vi "Read Number of Crossover Points.vi"(8 "error in (no error)":errorcluster, 11 "N-Point Crossover in":refnum<class "N-Point Crossover.lvclass">) -> (0 "error out":errorcluster, 2 "X-Point":T1, 3 "N-Point Crossover out":refnum<class "N-Point Crossover.lvclass">)   [LabVIEW 2016, in "N-Point Crossover.lvclass"]
uses:
  N-Point Crossover.lvclass
  _Typedefs/X-Point Crossover.ctl
  N-Point Crossover.lvclass/N-Point Crossover.ctl
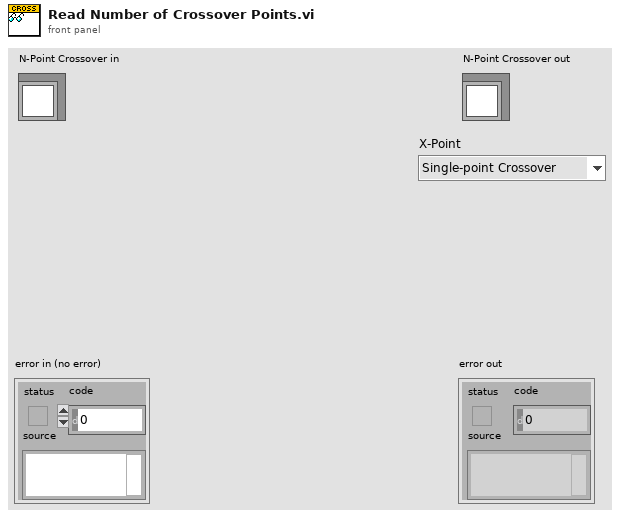
[diagram p1: front panel]
types:
  T1 = typedef "N-Point Crossover.lvclass/X-Point Crossover.ctl" = enum16{"Single-point Crossover", "Dual-point Crossover"}
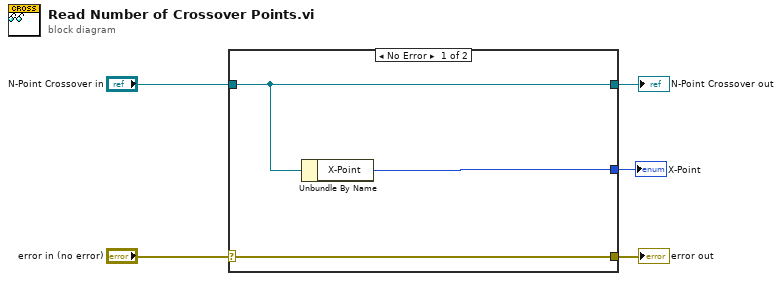
[diagram p0: block diagram]
diagram:
  n1 = case shown="No Error" "error in (no error)" {
    selector: "error in (no error)" -> [w8 w9]
    tunnel: [w8 w9] -> w4
    tunnel: [w7 w10] -> w2
    tunnel: "N-Point Crossover in" -> [w7 w10]
    tunnel: [w6 _] -> w1
    frame No Error {
      n2 = Unbundle By Name(w7) -> ("X-Point"=w6:T1)
    }
    frame Error {
    }
  }
  "error out" <- w4
  "N-Point Crossover out" <- w2
  "X-Point" <- w1
